vi "Execute_Circle_v2.vi"(0 "x-disp inp.":sgl[](array[numeric]), 1 "y-disp inp.":sgl[](array[numeric]), 2 "Resolution":u16=20, 3 "Speed":i32=200, 4 "Current (mA)":dbl, 5 "Laser GPIB":u8=10 max=100, 6 "Motor GPIB":u8=6) -> ()   [LabVIEW 2010]
uses:
  <vilib>/express/express arith-compare/Formula/XNode/ExpressFormulaBlockNode.xnode
panel:
  out "Dummy":string
  out "y-speed":sgl
  out "y-dist":sgl
  out "y-LR":bool
  out "x-speed":sgl
  out "x-dist":sgl
  out "x-LR":bool=TRUE
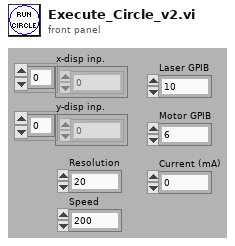
[diagram p1: front panel]
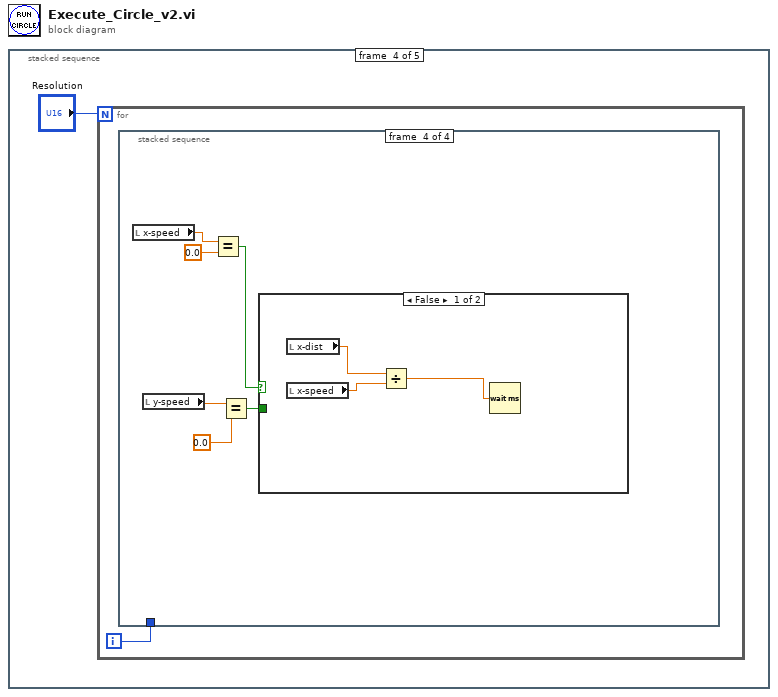
[diagram p0: block diagram]
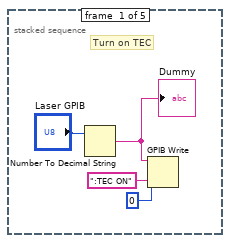
[diagram p2: hidden frame]
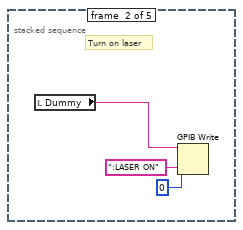
[diagram p3: hidden frame]
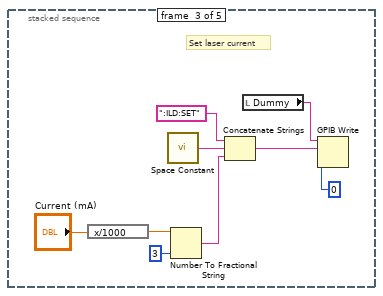
[diagram p4: hidden frame]
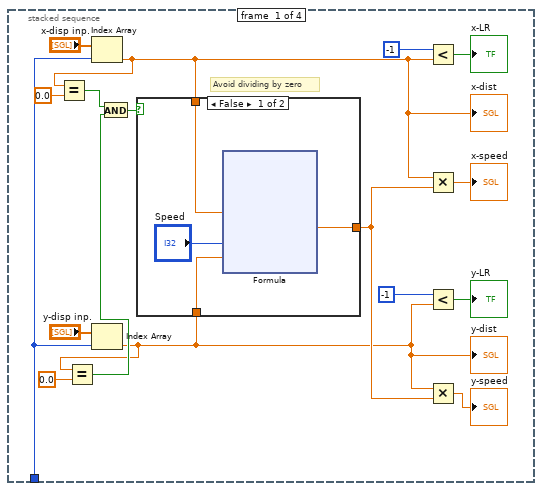
[diagram p5: hidden frame]
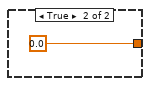
[diagram p6: hidden frame]
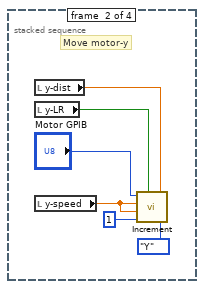
[diagram p7: hidden frame]
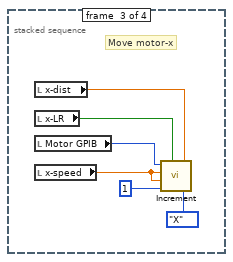
[diagram p8: hidden frame]
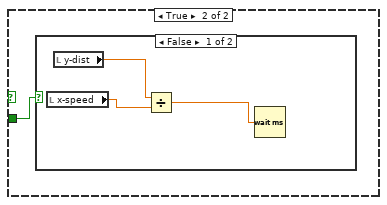
[diagram p9: hidden frame]
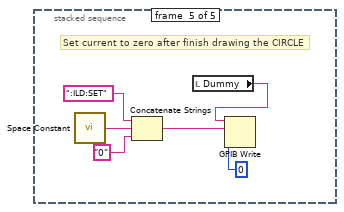
[diagram p11: hidden frame]
diagram:
  n1 = stacked-sequence {
    frame #0 {
      # "Turn on TEC"
      n2 = Number To Decimal String(number="Laser GPIB") -> (decimal integer string=w1:string)  [unwired: 1 in]
      "Dummy" <- w1
      n3 = GPIB Write(0:w1, 1:":TEC ON" ("data"), 2:i16 0 ("mode (0)")) -> ()  [unwired: 2 in, 2 out]
    }
    frame #1 {
      # "Turn on laser"
      n4 = local read "Dummy"() -> (w5:string)
      n5 = GPIB Write(0:w5, 1:":LASER ON" ("data"), 2:i16 0 ("mode (0)")) -> ()  [unwired: 2 in, 2 out]
    }
    frame #2 {
      # "Set laser current"
      n6 = expression code="x/1000"("Current (mA)") -> (w12:dbl)
      n7 = call <vilib>:"Space Constant.vi"() -> ("String"=w14:string)
      n8 = Number To Fractional String(number=w12, precision (6)=i16 3) -> (F-format string=w9:string)  [unwired: 2 in]
      n9 = Concatenate Strings(":ILD:SET", w14, w9) -> (w13:string)
      n10 = local read "Dummy"() -> (w8:string)
      n11 = GPIB Write(0:w8, 1:w13, 2:i16 0 ("mode (0)")) -> ()  [unwired: 2 in, 2 out]
    }
    frame #3 {
      n12 = for {
        N: "Resolution" -> [_]
        i -> [w18]
        n13 = stacked-sequence {
          tunnel: w18 -> [w31 _ _ _]
          frame #0 {
            # "Avoid dividing by zero"
            n14 = Index Array(array="x-disp inp.", index=w31) -> (element=w23:sgl)
            "x-dist" <- w23
            n15 = Equal?(x=w23, y=sgl 0.0) -> (x = y?=w28:bool)
            n16 = Index Array(array="y-disp inp.", index=w31) -> (element=w20:sgl)
            "y-dist" <- w20
            n17 = Equal?(x=w20, y=sgl 0.0) -> (x = y?=w27:bool)
            n18 = And(x=w28, y=w27) -> (x .and. y?=w26:bool)
            n19 = case shown="False" w26 {
              tunnel: [w36 sgl 0.0] -> w25
              tunnel: w23 -> [w38 _]
              tunnel: w20 -> [w37 _]
              frame False {
                n20 = xnode "Formula"("X1"=w38, "X2"="Speed", "X3"=w37) -> ("Result"=w36:sgl)  [unwired: 1 in, 1 out]
              }
              frame True {
              }
            }
            n21 = Less?(x=-1, y=w23) -> (x < y?=→"x-LR":bool)
            n22 = Multiply(x=w23, y=w25) -> (x*y=→"x-speed":sgl)
            n23 = Less?(x=-1, y=w20) -> (x < y?=→"y-LR":bool)
            n24 = Multiply(x=w20, y=w25) -> (x*y=→"y-speed":sgl)
          }
          frame #1 {
            # "Move motor-y"
            n25 = local read "y-dist"() -> (w53:sgl)
            n26 = local read "y-LR"() -> (w54:bool)
            n27 = local read "y-speed"() -> (w55:sgl)
            n28 = call "Increment.vi"("GPIB_Addr"="Motor GPIB", "F Speed"=w55, "L Speed"=w55, "Rate"=u16 1, "CCW 3"=w54, "Distance"=w53, "Axis"=enum16{"X", "Y", "Z", "U", "V", "W"}."Y") -> ()
          }
          frame #2 {
            # "Move motor-x"
            n29 = local read "x-dist"() -> (w61:sgl)
            n30 = local read "x-LR"() -> (w60:bool)
            n31 = local read "Motor GPIB"() -> (w64:u8)
            n32 = local read "x-speed"() -> (w59:sgl)
            n33 = call "Increment.vi"("GPIB_Addr"=w64, "F Speed"=w59, "L Speed"=w59, "Rate"=u16 1, "CCW 3"=w60, "Distance"=w61, "Axis"=enum16{"X", "Y", "Z", "U", "V", "W"}."X") -> ()
          }
          frame #3 {
            n34 = local read "x-speed"() -> (w70:sgl)
            n35 = local read "y-speed"() -> (w66:sgl)
            n36 = Equal?(x=w70, y=sgl 0.0) -> (x = y?=w68:bool)
            n37 = Equal?(x=w66, y=0.0) -> (x = y?=w65:bool)
            n38 = case shown="False" w68 {
              tunnel: w65 -> [_ w74]
              frame False {
                n39 = local read "x-dist"() -> (w73:sgl)
                n40 = local read "x-speed"() -> (w72:sgl)
                n41 = Divide(x=w73, y=w72) -> (x/y=w71:sgl)
                n42 = Wait (ms)(milliseconds to wait=w71) -> ()  [unwired: 1 out]
              }
              frame True {
                n43 = case shown="False" w74 {
                  frame False {
                    n44 = local read "x-speed"() -> (w75:sgl)
                    n45 = local read "y-dist"() -> (w76:sgl)
                    n46 = Divide(x=w76, y=w75) -> (x/y=w77:sgl)
                    n47 = Wait (ms)(milliseconds to wait=w77) -> ()  [unwired: 1 out]
                  }
                  frame True {
                  }
                }
              }
            }
          }
        }
      }
    }
    frame #4 {
      # "Set current to zero after finish drawing the CIRCLE"
      n48 = call <vilib>:"Space Constant.vi"() -> ("String"=w80:string)
      n49 = Concatenate Strings(":ILD:SET", w80, "0" ("string")) -> (w81:string)
      n50 = local read "Dummy"() -> (w82:string)
      n51 = GPIB Write(0:w82, 1:w81, 2:i16 0 ("mode (0)")) -> ()  [unwired: 2 in, 2 out]
    }
  }
